vi "Max_Min_gate_conversion.vi"(10 "Min":dbl, 11 "Max":dbl) -> (2 "offset":dbl, 3 "Amplitude":dbl)   [LabVIEW 2019, in "SMO.Transport.lvclass"]
uses:
  SMO.Transport.lvclass
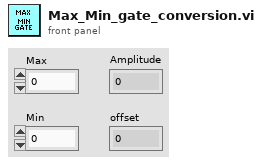
[diagram p1: front panel]
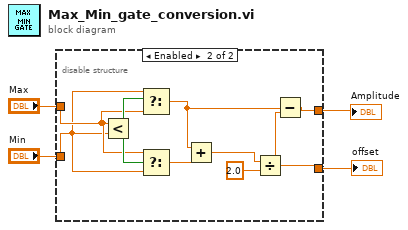
[diagram p0: block diagram]
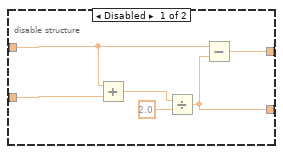
[diagram p2: hidden frame]
diagram:
  n1 = disable-structure shown="Enabled" {
    disable-tunnel: "Max" -> [w8 w14]
    disable-tunnel: "Min" -> [w7 w13]
    disable-tunnel: [w6 w12] -> w2
    disable-tunnel: [w5 w11] -> w1
    frame Disabled {
      n2 = Add(x=w8, y=w7) -> (x+y=w10:dbl)
      n3 = Divide(x=w10, y=2.0) -> (x/y=w5:dbl)
      n4 = Subtract(x=w8, y=w5) -> (x-y=w6:dbl)
    }
    frame Enabled {
      n5 = Less?(x=w14, y=w13) -> (x < y?=w17:bool)
      n6 = Select(t=w13, s=w17, f=w14) -> (s? t:f=w18:dbl)
      n7 = Select(t=w14, s=w17, f=w13) -> (s? t:f=w19:dbl)
      n8 = Add(x=w18, y=w19) -> (x+y=w15:dbl)
      n9 = Divide(x=w15, y=2.0) -> (x/y=w11:dbl)
      n10 = Subtract(x=w18, y=w11) -> (x-y=w12:dbl)
    }
  }
  "Amplitude" <- w2
  "offset" <- w1
